vi "Lab Panel V6.00.vi"() -> ()   [LabVIEW 2017] (continued)
                            n2540 = Build Array(w4644) -> (w4630:dbl[])
                            n2541 = Build Array(w4639) -> (w4635:dbl[])
                            n2542 = Build Array(w4637) -> (w4634:dbl[])
                            n2543 = Build Array(w4642) -> (w4629:dbl[])
                            n2544 = Build Array("AMPS ON", "AMPS OFF", "VOLTS", "PF", "TEMP Live", "TEMP Neut", "CYCLE") -> (w4612:string[])
                            n2545 = Bundle By Name("Y"=w4635, "t0"=w4628) -> (w4627:waveform(dbl))  [unwired: 1 in]
                            n2546 = Bundle By Name("Y"=w4634, "t0"=w4628) -> (w4626:waveform(dbl))  [unwired: 1 in]
                            n2547 = Bundle By Name("Y"=w4633, "t0"=w4628) -> (w4625:waveform(dbl))  [unwired: 1 in]
                            n2548 = Bundle By Name("Y"=w4632, "t0"=w4628) -> (w4624:waveform(dbl))  [unwired: 1 in]
                            n2549 = Bundle By Name("Y"=w4631, "t0"=w4628) -> (w4623:waveform(dbl))  [unwired: 1 in]
                            n2550 = Bundle By Name("Y"=w4630, "t0"=w4628) -> (w4622:waveform(dbl))  [unwired: 1 in]
                            n2551 = Bundle By Name("Y"=w4629, "t0"=w4628) -> (w4621:waveform(dbl))  [unwired: 1 in]
                            n2552 = Build Array(w4627, w4626, w4625, w4624, w4623, w4622, w4621) -> (w4620:waveform(dbl)[])
                            n2553 = TDMS Write(0:w4641, 5:"TEST VALUES", 7:w4612, 9:w4620) -> (4:w4611:refnum<k34>, 6:w4610:string, 15:w4609:errorcluster)  [unwired: 2 in, 1 out]
                            n2554 = TDMS Write(0:w4611, 5:w4610, 7:"TIME", 9:w4607, 11:w4609) -> (15:w4606:errorcluster)  [unwired: 1 in, 3 out]
                            n2555 = local write "data file error"(w4606) -> ()
                          }
                        }
                      }
                    }
                  }
                }
              }
              frame #8 {
                n2556 = case shown="True" w4645 {
                  tunnel: w4649 -> [_ w4654]
                  tunnel: w4648 -> [_ w4653]
                  tunnel: w4647 -> [_ w4651]
                  tunnel: w4646 -> [_ w4650]
                  frame False {
                  }
                  frame True {
                    n2557 = local read "DISP LAB05-1"() -> (w4655:T4)
                    n2558 = local read "SIG LAB05-1"() -> (w4656:T2)
                    n2559 = local read "ON L05-1"() -> (w4652:cluster{"amps":dbl, "volts":dbl, "pf":dbl})
                    n2560 = Unbundle(w4656) -> ("AMPS"=w4662:dbl, "VOLTS"=w4660:dbl, "PF"=w4659:dbl, "Tmp Live"=w4658:dbl, "Tmp Neut"=w4661:dbl)
                    n2561 = Unbundle(w4655) -> ("CYCLE"=w4657:dbl)  [unwired: 2 out]
                    n2562 = stacked-sequence {
                      tunnel: w4662 -> [w4666 w4685]
                      tunnel: w4661 -> [_ w4684]
                      tunnel: w4660 -> [w4665 w4683]
                      tunnel: w4659 -> [w4664 w4682]
                      tunnel: w4658 -> [_ w4681]
                      tunnel: w4657 -> [_ w4680]
                      tunnel: w4654 -> [_ w4679]
                      tunnel: w4653 -> [w4667 _]
                      tunnel: w4652 -> [w4663 w4677]
                      tunnel: w4651 -> [_ w4678]
                      tunnel: w4650 -> [_ w4673]
                      frame #0 {
                        n2563 = case shown="True" w4667 {
                          tunnel: w4666 -> [_ w4672]
                          tunnel: w4665 -> [_ w4671]
                          tunnel: w4664 -> [_ w4670]
                          tunnel: w4663 -> [_ w4668]
                          frame False {
                          }
                          frame True {
                            n2564 = Bundle(cluster=w4668, "amps"=w4672, "volts"=w4671, "pf"=w4670) -> (w4669:cluster{"amps":dbl, "volts":dbl, "pf":dbl})
                            n2565 = local write "ON L05-1"(w4669) -> ()
                          }
                        }
                      }
                      frame #1 {
                        n2566 = Unbundle(w4677) -> ("amps"=w4676:dbl, "volts"=w4675:dbl, "pf"=w4674:dbl)
                        n2567 = case shown="True" w4678 {
                          tunnel: w4685 -> [_ w4717]
                          tunnel: w4684 -> [_ w4724]
                          tunnel: w4683 -> [_ _]
                          tunnel: w4682 -> [_ _]
                          tunnel: w4681 -> [_ w4723]
                          tunnel: w4680 -> [_ w4722]
                          tunnel: w4679 -> [_ w4687]
                          tunnel: w4676 -> [_ w4719]
                          tunnel: w4675 -> [_ w4718]
                          tunnel: w4674 -> [_ w4716]
                          tunnel: w4673 -> [_ w4708]
                          frame False {
                          }
                          frame True {
                            n2568 = local read "TDMS LAB05-1"() -> (w4721:refnum<k34>)
                            n2569 = Build Array(w4718) -> (w4713:dbl[])
                            n2570 = Build Array(w4716) -> (w4712:dbl[])
                            n2571 = Build Array(w4723) -> (w4711:dbl[])
                            n2572 = Build Array(w4724) -> (w4710:dbl[])
                            n2573 = Build Array(w4719) -> (w4715:dbl[])
                            n2574 = Build Array(w4717) -> (w4714:dbl[])
                            n2575 = Build Array(w4722) -> (w4709:dbl[])
                            n2576 = Build Array("AMPS ON", "AMPS OFF", "VOLTS", "PF", "TEMP Live", "TEMP Neut", "CYCLE") -> (w4692:string[])
                            n2577 = Bundle By Name("Y"=w4715, "t0"=w4708) -> (w4707:waveform(dbl))  [unwired: 1 in]
                            n2578 = Bundle By Name("Y"=w4714, "t0"=w4708) -> (w4706:waveform(dbl))  [unwired: 1 in]
                            n2579 = Bundle By Name("Y"=w4713, "t0"=w4708) -> (w4705:waveform(dbl))  [unwired: 1 in]
                            n2580 = Bundle By Name("Y"=w4712, "t0"=w4708) -> (w4704:waveform(dbl))  [unwired: 1 in]
                            n2581 = Bundle By Name("Y"=w4711, "t0"=w4708) -> (w4703:waveform(dbl))  [unwired: 1 in]
                            n2582 = Bundle By Name("Y"=w4710, "t0"=w4708) -> (w4702:waveform(dbl))  [unwired: 1 in]
                            n2583 = Bundle By Name("Y"=w4709, "t0"=w4708) -> (w4701:waveform(dbl))  [unwired: 1 in]
                            n2584 = Build Array(w4707, w4706, w4705, w4704, w4703, w4702, w4701) -> (w4700:waveform(dbl)[])
                            n2585 = TDMS Write(0:w4721, 5:"TEST VALUES", 7:w4692, 9:w4700) -> (4:w4691:refnum<k34>, 6:w4690:string, 15:w4689:errorcluster)  [unwired: 2 in, 1 out]
                            n2586 = TDMS Write(0:w4691, 5:w4690, 7:"TIME", 9:w4687, 11:w4689) -> (15:w4686:errorcluster)  [unwired: 1 in, 3 out]
                            n2587 = local write "data file error"(w4686) -> ()
                          }
                        }
                      }
                    }
                  }
                }
              }
              frame #9 {
                n2588 = case shown="True" w4725 {
                  tunnel: w4729 -> [_ w4734]
                  tunnel: w4728 -> [_ w4733]
                  tunnel: w4727 -> [_ w4731]
                  tunnel: w4726 -> [_ w4730]
                  frame False {
                  }
                  frame True {
                    n2589 = local read "DISP LAB05-2"() -> (w4735:T4)
                    n2590 = local read "SIG LAB05-2"() -> (w4736:T2)
                    n2591 = local read "ON L05-2"() -> (w4732:cluster{"amps":dbl, "volts":dbl, "pf":dbl})
                    n2592 = Unbundle(w4736) -> ("AMPS"=w4742:dbl, "VOLTS"=w4740:dbl, "PF"=w4739:dbl, "Tmp Live"=w4738:dbl, "Tmp Neut"=w4741:dbl)
                    n2593 = Unbundle(w4735) -> ("CYCLE"=w4737:dbl)  [unwired: 2 out]
                    n2594 = stacked-sequence {
                      tunnel: w4742 -> [w4746 w4765]
                      tunnel: w4741 -> [_ w4764]
                      tunnel: w4740 -> [w4745 w4763]
                      tunnel: w4739 -> [w4744 w4762]
                      tunnel: w4738 -> [_ w4761]
                      tunnel: w4737 -> [_ w4760]
                      tunnel: w4734 -> [_ w4759]
                      tunnel: w4733 -> [w4747 _]
                      tunnel: w4732 -> [w4743 w4757]
                      tunnel: w4731 -> [_ w4758]
                      tunnel: w4730 -> [_ w4753]
                      frame #0 {
                        n2595 = case shown="True" w4747 {
                          tunnel: w4746 -> [_ w4752]
                          tunnel: w4745 -> [_ w4751]
                          tunnel: w4744 -> [_ w4750]
                          tunnel: w4743 -> [_ w4748]
                          frame False {
                          }
                          frame True {
                            n2596 = Bundle(cluster=w4748, "amps"=w4752, "volts"=w4751, "pf"=w4750) -> (w4749:cluster{"amps":dbl, "volts":dbl, "pf":dbl})
                            n2597 = local write "ON L05-2"(w4749) -> ()
                          }
                        }
                      }
                      frame #1 {
                        n2598 = Unbundle(w4757) -> ("amps"=w4756:dbl, "volts"=w4755:dbl, "pf"=w4754:dbl)
                        n2599 = case shown="True" w4758 {
                          tunnel: w4765 -> [_ w4797]
                          tunnel: w4764 -> [_ w4804]
                          tunnel: w4763 -> [_ _]
                          tunnel: w4762 -> [_ _]
                          tunnel: w4761 -> [_ w4803]
                          tunnel: w4760 -> [_ w4802]
                          tunnel: w4759 -> [_ w4767]
                          tunnel: w4756 -> [_ w4799]
                          tunnel: w4755 -> [_ w4798]
                          tunnel: w4754 -> [_ w4796]
                          tunnel: w4753 -> [_ w4788]
                          frame False {
                          }
                          frame True {
                            n2600 = local read "TDMS LAB05-2"() -> (w4801:refnum<k34>)
                            n2601 = Build Array(w4798) -> (w4793:dbl[])
                            n2602 = Build Array(w4796) -> (w4792:dbl[])
                            n2603 = Build Array(w4803) -> (w4791:dbl[])
                            n2604 = Build Array(w4804) -> (w4790:dbl[])
                            n2605 = Build Array(w4799) -> (w4795:dbl[])
                            n2606 = Build Array(w4797) -> (w4794:dbl[])
                            n2607 = Build Array(w4802) -> (w4789:dbl[])
                            n2608 = Build Array("AMPS ON", "AMPS OFF", "VOLTS", "PF", "TEMP Live", "TEMP Neut", "CYCLE") -> (w4772:string[])
                            n2609 = Bundle By Name("Y"=w4795, "t0"=w4788) -> (w4787:waveform(dbl))  [unwired: 1 in]
                            n2610 = Bundle By Name("Y"=w4794, "t0"=w4788) -> (w4786:waveform(dbl))  [unwired: 1 in]
                            n2611 = Bundle By Name("Y"=w4793, "t0"=w4788) -> (w4785:waveform(dbl))  [unwired: 1 in]
                            n2612 = Bundle By Name("Y"=w4792, "t0"=w4788) -> (w4784:waveform(dbl))  [unwired: 1 in]
                            n2613 = Bundle By Name("Y"=w4791, "t0"=w4788) -> (w4783:waveform(dbl))  [unwired: 1 in]
                            n2614 = Bundle By Name("Y"=w4790, "t0"=w4788) -> (w4782:waveform(dbl))  [unwired: 1 in]
                            n2615 = Bundle By Name("Y"=w4789, "t0"=w4788) -> (w4781:waveform(dbl))  [unwired: 1 in]
                            n2616 = Build Array(w4787, w4786, w4785, w4784, w4783, w4782, w4781) -> (w4780:waveform(dbl)[])
                            n2617 = TDMS Write(0:w4801, 5:"TEST VALUES", 7:w4772, 9:w4780) -> (4:w4771:refnum<k34>, 6:w4770:string, 15:w4769:errorcluster)  [unwired: 2 in, 1 out]
                            n2618 = TDMS Write(0:w4771, 5:w4770, 7:"TIME", 9:w4767, 11:w4769) -> (15:w4766:errorcluster)  [unwired: 1 in, 3 out]
                            n2619 = local write "data file error"(w4766) -> ()
                          }
                        }
                      }
                    }
                  }
                }
              }
            }
          }
          frame #15 {
            # "display test values on chart"
            n2620 = local read "jig cycle"() -> (w4809:dbl)
            n2621 = local read "on loops"() -> (w4811:dbl)
            n2622 = Add(x=w4811, y=4) -> (x+y=w4808:dbl)
            n2623 = Equal?(x=w4809, y=3) -> (x = y?=w4807:bool)
            n2624 = Equal?(x=w4809, y=w4808) -> (x = y?=w4806:bool)
            n2625 = Or(x=w4807, y=w4806) -> (x .or. y?=w4805:bool)
            "graph flag" <- w4805
            n2626 = global write "Global display 3.vi" "graph flag"(w4805) -> ()
            n2627 = case shown="True" w4805 {
              frame False {
              }
              frame True {
                n2628 = local read "SIG LAB05-1"() -> (w4854:T2)
                n2629 = local read "SIG LAB04-2"() -> (w4855:T2)
                n2630 = local read "SIG LAB05-2"() -> (w4853:T2)
                n2631 = local read "SIG LAB04-1"() -> (w4856:T2)
                n2632 = local read "SIG LAB01-1"() -> (w4862:T2)
                n2633 = local read "SIG LAB03-1"() -> (w4858:T2)
                n2634 = local read "SIG LAB03-2"() -> (w4857:T2)
                n2635 = local read "SIG LAB02-2"() -> (w4859:T2)
                n2636 = local read "SIG LAB02-1"() -> (w4860:T2)
                n2637 = local read "SIG LAB01-2"() -> (w4861:T2)
                n2638 = Unbundle By Name(w4862) -> ("AMPS"=w4852:dbl, "VOLTS"=w4842:dbl, "Tmp Live"=w4832:dbl, "Tmp Neut"=w4822:dbl)
                n2639 = Unbundle(w4855) -> ("AMPS"=w4845:dbl, "VOLTS"=w4835:dbl, "Tmp Live"=w4825:dbl, "Tmp Neut"=w4815:dbl)  [unwired: 1 out]
                n2640 = Unbundle(w4854) -> ("AMPS"=w4844:dbl, "VOLTS"=w4834:dbl, "Tmp Live"=w4824:dbl, "Tmp Neut"=w4814:dbl)  [unwired: 1 out]
                n2641 = Unbundle(w4853) -> ("AMPS"=w4843:dbl, "VOLTS"=w4833:dbl, "Tmp Live"=w4823:dbl, "Tmp Neut"=w4813:dbl)  [unwired: 1 out]
                n2642 = Unbundle(w4856) -> ("AMPS"=w4846:dbl, "VOLTS"=w4836:dbl, "Tmp Live"=w4826:dbl, "Tmp Neut"=w4816:dbl)  [unwired: 1 out]
                n2643 = Unbundle(w4857) -> ("AMPS"=w4847:dbl, "VOLTS"=w4837:dbl, "Tmp Live"=w4827:dbl, "Tmp Neut"=w4817:dbl)  [unwired: 1 out]
                n2644 = Unbundle(w4858) -> ("AMPS"=w4848:dbl, "VOLTS"=w4838:dbl, "Tmp Live"=w4828:dbl, "Tmp Neut"=w4818:dbl)  [unwired: 1 out]
                n2645 = Unbundle(w4859) -> ("AMPS"=w4849:dbl, "VOLTS"=w4839:dbl, "Tmp Live"=w4829:dbl, "Tmp Neut"=w4819:dbl)  [unwired: 1 out]
                n2646 = Unbundle(w4860) -> ("AMPS"=w4850:dbl, "VOLTS"=w4840:dbl, "Tmp Live"=w4830:dbl, "Tmp Neut"=w4820:dbl)  [unwired: 1 out]
                n2647 = Unbundle(w4861) -> ("AMPS"=w4851:dbl, "VOLTS"=w4841:dbl, "Tmp Live"=w4831:dbl, "Tmp Neut"=w4821:dbl)  [unwired: 1 out]
                n2648 = stacked-sequence {
                  tunnel: w4852 -> [w4894 _ _]
                  tunnel: w4851 -> [w4893 _ _]
                  tunnel: w4850 -> [w4884 _ _]
                  tunnel: w4849 -> [w4883 _ _]
                  tunnel: w4848 -> [w4873 _ _]
                  tunnel: w4847 -> [w4872 _ _]
                  tunnel: w4846 -> [_ w4917 _]
                  tunnel: w4845 -> [_ w4916 _]
                  tunnel: w4844 -> [_ w4906 _]
                  tunnel: w4843 -> [_ w4905 _]
                  tunnel: w4842 -> [w4891 _ _]
                  tunnel: w4841 -> [w4890 _ _]
                  tunnel: w4840 -> [w4881 _ _]
                  tunnel: w4839 -> [w4880 _ _]
                  tunnel: w4838 -> [w4871 _ _]
                  tunnel: w4837 -> [w4870 _ _]
                  tunnel: w4836 -> [_ w4915 _]
                  tunnel: w4835 -> [_ w4914 _]
                  tunnel: w4834 -> [_ w4904 _]
                  tunnel: w4833 -> [_ w4903 _]
                  tunnel: w4832 -> [w4888 _ _]
                  tunnel: w4831 -> [w4886 _ _]
                  tunnel: w4830 -> [w4877 _ _]
                  tunnel: w4829 -> [w4875 _ _]
                  tunnel: w4828 -> [w4869 _ _]
                  tunnel: w4827 -> [w4867 _ _]
                  tunnel: w4826 -> [_ w4913 _]
                  tunnel: w4825 -> [_ w4911 _]
                  tunnel: w4824 -> [_ w4902 _]
                  tunnel: w4823 -> [_ w4900 _]
                  tunnel: w4822 -> [w4887 _ _]
                  tunnel: w4821 -> [w4885 _ _]
                  tunnel: w4820 -> [w4876 _ _]
                  tunnel: w4819 -> [w4874 _ _]
                  tunnel: w4818 -> [w4868 _ _]
                  tunnel: w4817 -> [w4866 _ _]
                  tunnel: w4816 -> [_ w4912 _]
                  tunnel: w4815 -> [_ w4910 _]
                  tunnel: w4814 -> [_ w4901 _]
                  tunnel: w4813 -> [_ w4899 _]
                  frame #0 {
                    n2649 = Merge Signals(w4894, w4893) -> (→"LAB01 AMPS":dynamicdata)
                    n2650 = Merge Signals(w4891, w4890) -> (→"LAB01 VOLTS":dynamicdata)
                    n2651 = Merge Signals(w4871, w4870) -> (→"LAB03 VOLTS":dynamicdata)
                    n2652 = Merge Signals(w4888, w4887, w4886, w4885) -> (→"LAB01 deg C":dynamicdata)
                    n2653 = Merge Signals(w4884, w4883) -> (→"LAB02 AMPS":dynamicdata)
                    n2654 = Merge Signals(w4877, w4876, w4875, w4874) -> (→"LAB02 deg C":dynamicdata)
                    n2655 = Merge Signals(w4869, w4868, w4867, w4866) -> (→"LAB03 deg C":dynamicdata)
                    n2656 = Merge Signals(w4881, w4880) -> (→"LAB02 VOLTS":dynamicdata)
                    n2657 = Merge Signals(w4873, w4872) -> (→"LAB03 AMPS":dynamicdata)
                  }
                  frame #1 {
                    n2658 = Merge Signals(w4904, w4903) -> (→"LAB05 VOLTS":dynamicdata)
                    n2659 = Merge Signals(w4917, w4916) -> (→"LAB04 AMPS":dynamicdata)
                    n2660 = Merge Signals(w4906, w4905) -> (→"LAB05 AMPS":dynamicdata)
                    n2661 = Merge Signals(w4902, w4901, w4900, w4899) -> (→"LAB05 deg C":dynamicdata)
                    n2662 = Merge Signals(w4913, w4912, w4911, w4910) -> (→"LAB04 deg C":dynamicdata)
                    n2663 = Merge Signals(w4915, w4914) -> (→"LAB04 VOLTS":dynamicdata)
                  }
                  frame #2 {
                    n2664 = local read "LAB05 VOLTS"() -> (w4925:dynamicdata)
                    n2665 = local read "LAB04 VOLTS"() -> (w4926:dynamicdata)
                    n2666 = local read "LAB05 AMPS"() -> (w4931:dynamicdata)
                    n2667 = local read "LAB02 VOLTS"() -> (w4928:dynamicdata)
                    n2668 = local read "LAB03 VOLTS"() -> (w4927:dynamicdata)
                    n2669 = local read "LAB01 VOLTS"() -> (w4929:dynamicdata)
                    n2670 = local read "LAB04 AMPS"() -> (w4932:dynamicdata)
                    n2671 = local read "LAB03 AMPS"() -> (w4933:dynamicdata)
                    n2672 = local read "LAB03 deg C"() -> (w4921:dynamicdata)
                    n2673 = local read "LAB02 AMPS"() -> (w4934:dynamicdata)
                    n2674 = local read "LAB04 deg C"() -> (w4920:dynamicdata)
                    n2675 = local read "LAB05 deg C"() -> (w4919:dynamicdata)
                    n2676 = local read "LAB02 deg C"() -> (w4922:dynamicdata)
                    n2677 = local read "LAB01 deg C"() -> (w4923:dynamicdata)
                    n2678 = local read "LAB01 AMPS"() -> (w4935:dynamicdata)
                    n2679 = Merge Signals(w4923, w4922, w4921, w4920, w4919) -> (w4918:dynamicdata)
                    n2680 = Merge Signals(w4935, w4934, w4933, w4932, w4931) -> (w4930:dynamicdata)
                    n2681 = Merge Signals(w4929, w4928, w4927, w4926, w4925) -> (w4924:dynamicdata)
                    n2682 = global write "Global display 3.vi" "graph volts"(w4924) -> ()
                    n2683 = global write "Global display 3.vi" "graph deg C"(w4918) -> ()
                    n2684 = global write "Global display 3.vi" "graph amps"(w4930) -> ()
                  }
                }
              }
            }
          }
          frame #16 {
            # "check for amps fail"
            # "check for cycle test & temperature rise fail conditions"
            n2685 = local read "on loops"() -> (w4962:dbl)
            n2686 = local read "jig cycle"() -> (w4959:dbl)
            n2687 = Add(x=w4962, y=5.0) -> (x+y=w4960:dbl)
            n2688 = Equal?(x=w4959, y=w4960) -> (x = y?=w4955:bool)
            n2689 = local read "jig cycle"() -> (w4964:dbl)
            n2690 = Equal?(x=w4964, y=3.0) -> (x = y?=w4957:bool)
            n2691 = local read "Fail Loops"() -> (w4936:dbl)
            n2692 = stacked-sequence {
              tunnel: w4958 -> [w4967 _ _ _ _ _ _ _ _ _]
              tunnel: w4957 -> [w4968 w4988 w5008 w5028 w5048 w5068 w5088 w5108 w5128 w5148]
              tunnel: w4956 -> [w4965 _ _ _ _ _ _ _ _ _]
              tunnel: w4955 -> [w4966 w4987 w5007 w5027 w5047 w5067 w5087 w5107 w5127 w5147]
              tunnel: w4954 -> [_ w4986 _ _ _ _ _ _ _ _]
              tunnel: w4953 -> [_ w4985 _ _ _ _ _ _ _ _]
              tunnel: w4952 -> [_ _ w5006 _ _ _ _ _ _ _]
              tunnel: w4951 -> [_ _ w5005 _ _ _ _ _ _ _]
              tunnel: w4950 -> [_ _ _ w5026 _ _ _ _ _ _]
              tunnel: w4949 -> [_ _ _ w5025 _ _ _ _ _ _]
              tunnel: w4948 -> [_ _ _ _ w5046 _ _ _ _ _]
              tunnel: w4947 -> [_ _ _ _ w5045 _ _ _ _ _]
              tunnel: w4946 -> [_ _ _ _ _ w5066 _ _ _ _]
              tunnel: w4945 -> [_ _ _ _ _ w5065 _ _ _ _]
              tunnel: w4944 -> [_ _ _ _ _ _ w5086 _ _ _]
              tunnel: w4943 -> [_ _ _ _ _ _ w5085 _ _ _]
              tunnel: w4942 -> [_ _ _ _ _ _ _ w5106 _ _]
              tunnel: w4941 -> [_ _ _ _ _ _ _ w5105 _ _]
              tunnel: w4940 -> [_ _ _ _ _ _ _ _ w5126 _]
              tunnel: w4939 -> [_ _ _ _ _ _ _ _ w5125 _]
              tunnel: w4938 -> [_ _ _ _ _ _ _ _ _ w5146]
              tunnel: w4937 -> [_ _ _ _ _ _ _ _ _ w5145]
              frame #0 {
                # "LAB01-1"
                n2693 = case shown="True" w4965 {
                  tunnel: w4968 -> [_ w4981]
                  tunnel: w4967 -> [_ w4978]
                  tunnel: w4966 -> [_ w4977]
                  frame False {
                  }
                  frame True {
                    n2694 = local read "TEMP START LAB01-1"() -> (w4983:cluster{"TL":dbl, "TN":dbl})
                    n2695 = local read "RESULT LAB01-1"() -> (w4972:bool)
                    n2696 = local read "FAIL LAB01-1"() -> (w4975:cluster{"LO":dbl, "HI":dbl})
                    n2697 = local read "TDMS LAB01-1"() -> (w4982:refnum<k34>)
                    n2698 = local read "SET LAB01-1"() -> (w4979:T6)
                    n2699 = local read "DISP LAB01-1"() -> (w4980:T4)
                    n2700 = local read "SIG LAB01-1"() -> (w4984:T2)
                    n2701 = Bundle("FAIL LAB01-1"=w4975, "SIG LAB01-1"=w4984, "TEMP START LAB01-1"=w4983, "DISP LAB01-1"=w4980, "SET LAB01-1"=w4979, "TDMS LAB01-1"=w4982) -> (w4969:T36)  [unwired: 1 in]
                    n2702 = call "sub vi - cycle&temp fail v7.vi"("Amps Lo?"=w4981, "Input Cluster"=w4969, "SELECT"=w4978, "Amps Hi?"=w4977, "Result In"=w4972) -> ("(FAIL) out"=w4974:cluster{"FAIL LO":dbl, "FAIL HI":dbl}, "(DISP) out"=w4970:T4, "T-RISE"=w4971:cluster{"T-RISE (L)":dbl, "T-RISE (N)":dbl}, "Result Out"=w4973:bool, "file error"=w4976:errorcluster)  [unwired: 10 in]
                    n2703 = local write "TEMP RISE LAB01-1"(w4971) -> ()
                    n2704 = local write "FAIL LAB01-1"(w4974) -> ()
                    n2705 = local write "DISP LAB01-1"(w4970) -> ()
                    n2706 = local write "RESULT LAB01-1"(w4973) -> ()
                    n2707 = local write "data file error"(w4976) -> ()
                  }
                }
              }
              frame #1 {
                # "LAB01-2"
                n2708 = case shown="True" w4986 {
                  tunnel: w4988 -> [_ w5001]
                  tunnel: w4985 -> [_ w4998]
                  tunnel: w4987 -> [_ w4997]
                  frame False {
                  }
                  frame True {
                    n2709 = local read "TEMP START LAB01-2"() -> (w5003:cluster{"TL":dbl, "TN":dbl})
                    n2710 = local read "FAIL LAB01-2"() -> (w4994:cluster{"LO":dbl, "HI":dbl})
                    n2711 = local read "TDMS LAB01-2"() -> (w5002:refnum<k34>)
                    n2712 = local read "SET LAB01-2"() -> (w4999:T5)
                    n2713 = local read "DISP LAB01-2"() -> (w5000:T4)
                    n2714 = local read "RESULT LAB01-2"() -> (w4991:bool)
                    n2715 = local read "SIG LAB01-2"() -> (w5004:T2)
                    n2716 = Bundle("FAIL LAB01-2"=w4994, "SIG LAB01-2"=w5004, "TEMP START LAB01-2"=w5003, "DISP LAB01-2"=w5000, "SET LAB01-2"=w4999, "TDMS LAB01-2"=w5002) -> (w4989:T37)  [unwired: 1 in]
                    n2717 = call "sub vi - cycle&temp fail v7.vi"("Amps Lo?"=w5001, "Input Cluster"=w4989, "SELECT"=w4998, "Amps Hi?"=w4997, "Result In"=w4991) -> ("(FAIL) out"=w4993:cluster{"FAIL LO":dbl, "FAIL HI":dbl}, "(DISP) out"=w4996:T4, "T-RISE"=w4990:cluster{"T-RISE (L)":dbl, "T-RISE (N)":dbl}, "Result Out"=w4992:bool, "file error"=w4995:errorcluster)  [unwired: 10 in]
                    n2718 = local write "TEMP RISE LAB01-2"(w4990) -> ()
                    n2719 = local write "FAIL LAB01-2"(w4993) -> ()
                    n2720 = local write "DISP LAB01-2"(w4996) -> ()
                    n2721 = local write "RESULT LAB01-2"(w4992) -> ()
                    n2722 = local write "data file error"(w4995) -> ()
                  }
                }
              }
              frame #2 {
                # "LAB02-1"
                n2723 = case shown="True" w5006 {
                  tunnel: w5008 -> [_ w5021]
                  tunnel: w5005 -> [_ w5018]
                  tunnel: w5007 -> [_ w5017]
                  frame False {
                  }
                  frame True {
                    n2724 = local read "TEMP START LAB02-1"() -> (w5023:cluster{"TL":dbl, "TN":dbl})
                    n2725 = local read "FAIL LAB02-1"() -> (w5014:cluster{"LO":dbl, "HI":dbl})
                    n2726 = local read "TDMS LAB02-1"() -> (w5022:refnum<k34>)
                    n2727 = local read "SET LAB02-1"() -> (w5019:T5)
                    n2728 = local read "DISP LAB02-1"() -> (w5020:T4)
                    n2729 = local read "SIG LAB02-1"() -> (w5024:T2)
                    n2730 = local read "RESULT LAB02-1"() -> (w5011:bool)
                    n2731 = Bundle("FAIL LAB02-1"=w5014, "SIG LAB02-1"=w5024, "TEMP START LAB02-1"=w5023, "DISP LAB02-1"=w5020, "SET LAB02-1"=w5019, "TDMS LAB02-1"=w5022) -> (w5009:T38)  [unwired: 1 in]
                    n2732 = call "sub vi - cycle&temp fail v7.vi"("Amps Lo?"=w5021, "Input Cluster"=w5009, "SELECT"=w5018, "Amps Hi?"=w5017, "Result In"=w5011) -> ("(FAIL) out"=w5013:cluster{"FAIL LO":dbl, "FAIL HI":dbl}, "(DISP) out"=w5016:T4, "T-RISE"=w5010:cluster{"T-RISE (L)":dbl, "T-RISE (N)":dbl}, "Result Out"=w5012:bool, "file error"=w5015:errorcluster)  [unwired: 10 in]
                    n2733 = local write "TEMP RISE LAB02-1"(w5010) -> ()
                    n2734 = local write "FAIL LAB02-1"(w5013) -> ()
                    n2735 = local write "DISP LAB02-1"(w5016) -> ()
                    n2736 = local write "RESULT LAB02-1"(w5012) -> ()
                    n2737 = local write "data file error"(w5015) -> ()
                  }
                }
              }
              frame #3 {
                # "LAB02-2"
                n2738 = case shown="True" w5026 {
                  tunnel: w5028 -> [_ w5041]
                  tunnel: w5025 -> [_ w5038]
                  tunnel: w5027 -> [_ w5037]
                  frame False {
                  }
                  frame True {
                    n2739 = local read "TEMP START LAB02-2"() -> (w5043:cluster{"TL":dbl, "TN":dbl})
                    n2740 = local read "FAIL LAB02-2"() -> (w5034:cluster{"LO":dbl, "HI":dbl})
                    n2741 = local read "TDMS LAB02-2"() -> (w5042:refnum<k34>)
                    n2742 = local read "SET LAB02-2"() -> (w5039:T5)
                    n2743 = local read "DISP LAB02-2"() -> (w5040:T4)
                    n2744 = local read "SIG LAB02-2"() -> (w5044:T2)
                    n2745 = local read "RESULT LAB02-2"() -> (w5031:bool)
                    n2746 = Bundle("FAIL LAB02-2"=w5034, "SIG LAB02-2"=w5044, "TEMP START LAB02-2"=w5043, "DISP LAB02-2"=w5040, "SET LAB02-2"=w5039, "TDMS LAB02-2"=w5042) -> (w5029:T39)  [unwired: 1 in]
                    n2747 = call "sub vi - cycle&temp fail v7.vi"("Amps Lo?"=w5041, "Input Cluster"=w5029, "SELECT"=w5038, "Amps Hi?"=w5037, "Result In"=w5031) -> ("(FAIL) out"=w5033:cluster{"FAIL LO":dbl, "FAIL HI":dbl}, "(DISP) out"=w5036:T4, "T-RISE"=w5030:cluster{"T-RISE (L)":dbl, "T-RISE (N)":dbl}, "Result Out"=w5032:bool, "file error"=w5035:errorcluster)  [unwired: 10 in]
                    n2748 = local write "TEMP RISE LAB02-2"(w5030) -> ()
                    n2749 = local write "FAIL LAB02-2"(w5033) -> ()
                    n2750 = local write "DISP LAB02-2"(w5036) -> ()
                    n2751 = local write "RESULT LAB02-2"(w5032) -> ()
                    n2752 = local write "data file error"(w5035) -> ()
                  }
                }
              }
              frame #4 {
                # "LAB03-1"
                n2753 = case shown="True" w5046 {
                  tunnel: w5048 -> [_ w5061]
                  tunnel: w5045 -> [_ w5058]
                  tunnel: w5047 -> [_ w5057]
                  frame False {
                  }
                  frame True {
                    n2754 = local read "TEMP START LAB03-1"() -> (w5063:cluster{"TL":dbl, "TN":dbl})
                    n2755 = local read "FAIL LAB03-1"() -> (w5054:cluster{"LO":dbl, "HI":dbl})
                    n2756 = local read "TDMS LAB03-1"() -> (w5062:refnum<k34>)
                    n2757 = local read "SET LAB03-1"() -> (w5059:T5)
                    n2758 = local read "DISP LAB03-1"() -> (w5060:T4)
                    n2759 = local read "SIG LAB03-1"() -> (w5064:T2)
                    n2760 = local read "RESULT LAB03-1"() -> (w5051:bool)
                    n2761 = Bundle("FAIL LAB03-1"=w5054, "SIG LAB03-1"=w5064, "TEMP START LAB03-1"=w5063, "DISP LAB03-1"=w5060, "SET LAB03-1"=w5059, "TDMS LAB03-1"=w5062) -> (w5049:T40)  [unwired: 1 in]
                    n2762 = call "sub vi - cycle&temp fail v7.vi"("Amps Lo?"=w5061, "Input Cluster"=w5049, "SELECT"=w5058, "Amps Hi?"=w5057, "Result In"=w5051) -> ("(FAIL) out"=w5053:cluster{"FAIL LO":dbl, "FAIL HI":dbl}, "(DISP) out"=w5056:T4, "T-RISE"=w5050:cluster{"T-RISE (L)":dbl, "T-RISE (N)":dbl}, "Result Out"=w5052:bool, "file error"=w5055:errorcluster)  [unwired: 10 in]
                    n2763 = local write "TEMP RISE LAB03-1"(w5050) -> ()
                    n2764 = local write "FAIL LAB03-1"(w5053) -> ()
                    n2765 = local write "DISP LAB03-1"(w5056) -> ()
                    n2766 = local write "RESULT LAB03-1"(w5052) -> ()
                    n2767 = local write "data file error"(w5055) -> ()
                  }
                }
              }
              frame #5 {
                # "LAB03-2"
                n2768 = case shown="True" w5066 {
                  tunnel: w5068 -> [_ w5081]
                  tunnel: w5065 -> [_ w5078]
                  tunnel: w5067 -> [_ w5077]
                  frame False {
                  }
                  frame True {
                    n2769 = local read "TEMP START LAB03-2"() -> (w5083:cluster{"TL":dbl, "TN":dbl})
                    n2770 = local read "FAIL LAB03-2"() -> (w5074:cluster{"LO":dbl, "HI":dbl})
                    n2771 = local read "TDMS LAB03-2"() -> (w5082:refnum<k34>)
                    n2772 = local read "SET LAB03-2"() -> (w5079:T5)
                    n2773 = local read "DISP LAB03-2"() -> (w5080:T4)
                    n2774 = local read "RESULT LAB03-2"() -> (w5071:bool)
                    n2775 = local read "SIG LAB03-2"() -> (w5084:T2)
                    n2776 = Bundle("FAIL LAB03-2"=w5074, "SIG LAB03-2"=w5084, "TEMP START LAB03-2"=w5083, "DISP LAB03-2"=w5080, "SET LAB03-2"=w5079, "TDMS LAB03-2"=w5082) -> (w5069:T41)  [unwired: 1 in]
                    n2777 = call "sub vi - cycle&temp fail v7.vi"("Amps Lo?"=w5081, "Input Cluster"=w5069, "SELECT"=w5078, "Amps Hi?"=w5077, "Result In"=w5071) -> ("(FAIL) out"=w5073:cluster{"FAIL LO":dbl, "FAIL HI":dbl}, "(DISP) out"=w5076:T4, "T-RISE"=w5070:cluster{"T-RISE (L)":dbl, "T-RISE (N)":dbl}, "Result Out"=w5072:bool, "file error"=w5075:errorcluster)  [unwired: 10 in]
                    n2778 = local write "FAIL LAB03-2"(w5073) -> ()
                    n2779 = local write "TEMP RISE LAB03-2"(w5070) -> ()
                    n2780 = local write "DISP LAB03-2"(w5076) -> ()
                    n2781 = local write "RESULT LAB03-2"(w5072) -> ()
                    n2782 = local write "data file error"(w5075) -> ()
                  }
                }
              }
              frame #6 {
                # "LAB04-1"
                n2783 = case shown="True" w5086 {
                  tunnel: w5088 -> [_ w5101]
                  tunnel: w5085 -> [_ w5098]
                  tunnel: w5087 -> [_ w5097]
                  frame False {
                  }
                  frame True {
                    n2784 = local read "TEMP START LAB04-1"() -> (w5103:cluster{"TL":dbl, "TN":dbl})
                    n2785 = local read "FAIL LAB04-1"() -> (w5094:cluster{"LO":dbl, "HI":dbl})
                    n2786 = local read "TDMS LAB04-1"() -> (w5102:refnum<k34>)
                    n2787 = local read "SET LAB04-1"() -> (w5099:T5)
                    n2788 = local read "DISP LAB04-1"() -> (w5100:T4)
                    n2789 = local read "SIG LAB04-1"() -> (w5104:T2)
                    n2790 = local read "RESULT LAB04-1"() -> (w5091:bool)
                    n2791 = Bundle("FAIL LAB04-1"=w5094, "SIG LAB04-1"=w5104, "TEMP START LAB04-1"=w5103, "DISP LAB04-1"=w5100, "SET LAB04-1"=w5099, "TDMS LAB04-1"=w5102) -> (w5089:T42)  [unwired: 1 in]
                    n2792 = call "sub vi - cycle&temp fail v7.vi"("Amps Lo?"=w5101, "Input Cluster"=w5089, "SELECT"=w5098, "Amps Hi?"=w5097, "Result In"=w5091) -> ("(FAIL) out"=w5093:cluster{"FAIL LO":dbl, "FAIL HI":dbl}, "(DISP) out"=w5096:T4, "T-RISE"=w5090:cluster{"T-RISE (L)":dbl, "T-RISE (N)":dbl}, "Result Out"=w5092:bool, "file error"=w5095:errorcluster)  [unwired: 10 in]
                    n2793 = local write "TEMP RISE LAB04-1"(w5090) -> ()
                    n2794 = local write "FAIL LAB04-1"(w5093) -> ()
                    n2795 = local write "DISP LAB04-1"(w5096) -> ()
                    n2796 = local write "RESULT LAB04-1"(w5092) -> ()
                    n2797 = local write "data file error"(w5095) -> ()
                  }
                }
              }
              frame #7 {
                # "LAB04-2"
                n2798 = case shown="True" w5106 {
                  tunnel: w5108 -> [_ w5121]
                  tunnel: w5105 -> [_ w5118]
                  tunnel: w5107 -> [_ w5117]
                  frame False {
                  }
                  frame True {
                    n2799 = local read "TEMP START LAB04-2"() -> (w5123:cluster{"TL":dbl, "TN":dbl})
                    n2800 = local read "FAIL LAB04-2"() -> (w5114:cluster{"LO":dbl, "HI":dbl})
                    n2801 = local read "TDMS LAB04-2"() -> (w5122:refnum<k34>)
                    n2802 = local read "SET LAB04-2"() -> (w5119:T5)
                    n2803 = local read "DISP LAB04-2"() -> (w5120:T4)
                    n2804 = local read "SIG LAB04-2"() -> (w5124:T2)
                    n2805 = local read "RESULT LAB04-2"() -> (w5111:bool)
                    n2806 = Bundle("FAIL LAB04-2"=w5114, "SIG LAB04-2"=w5124, "TEMP START LAB04-2"=w5123, "DISP LAB04-2"=w5120, "SET LAB04-2"=w5119, "TDMS LAB04-2"=w5122) -> (w5109:T43)  [unwired: 1 in]
                    n2807 = call "sub vi - cycle&temp fail v7.vi"("Amps Lo?"=w5121, "Input Cluster"=w5109, "SELECT"=w5118, "Amps Hi?"=w5117, "Result In"=w5111) -> ("(FAIL) out"=w5113:cluster{"FAIL LO":dbl, "FAIL HI":dbl}, "(DISP) out"=w5116:T4, "T-RISE"=w5110:cluster{"T-RISE (L)":dbl, "T-RISE (N)":dbl}, "Result Out"=w5112:bool, "file error"=w5115:errorcluster)  [unwired: 10 in]
                    n2808 = local write "TEMP RISE LAB04-2"(w5110) -> ()
                    n2809 = local write "FAIL LAB04-2"(w5113) -> ()
                    n2810 = local write "DISP LAB04-2"(w5116) -> ()
                    n2811 = local write "RESULT LAB04-2"(w5112) -> ()
                    n2812 = local write "data file error"(w5115) -> ()
                  }
                }
              }
              frame #8 {
                # "LAB05-1"
                n2813 = case shown="True" w5126 {
                  tunnel: w5128 -> [_ w5141]
                  tunnel: w5125 -> [_ w5138]
                  tunnel: w5127 -> [_ w5137]
                  frame False {
                  }
                  frame True {
                    n2814 = local read "TEMP START LAB05-1"() -> (w5143:cluster{"TL":dbl, "TN":dbl})
                    n2815 = local read "FAIL LAB05-1"() -> (w5134:cluster{"LO":dbl, "HI":dbl})
                    n2816 = local read "TDMS LAB05-1"() -> (w5142:refnum<k34>)
                    n2817 = local read "SET LAB05-1"() -> (w5139:T5)
                    n2818 = local read "DISP LAB05-1"() -> (w5140:T4)
                    n2819 = local read "SIG LAB05-1"() -> (w5144:T2)
                    n2820 = local read "RESULT LAB05-1"() -> (w5131:bool)
                    n2821 = Bundle("FAIL LAB05-1"=w5134, "SIG LAB05-1"=w5144, "TEMP START LAB05-1"=w5143, "DISP LAB05-1"=w5140, "SET LAB05-1"=w5139, "TDMS LAB05-1"=w5142) -> (w5129:T44)  [unwired: 1 in]
                    n2822 = call "sub vi - cycle&temp fail v7.vi"("Amps Lo?"=w5141, "Input Cluster"=w5129, "SELECT"=w5138, "Amps Hi?"=w5137, "Result In"=w5131) -> ("(FAIL) out"=w5133:cluster{"FAIL LO":dbl, "FAIL HI":dbl}, "(DISP) out"=w5136:T4, "T-RISE"=w5130:cluster{"T-RISE (L)":dbl, "T-RISE (N)":dbl}, "Result Out"=w5132:bool, "file error"=w5135:errorcluster)  [unwired: 10 in]
                    n2823 = local write "TEMP RISE LAB05-1"(w5130) -> ()
                    n2824 = local write "FAIL LAB05-1"(w5133) -> ()
                    n2825 = local write "DISP LAB05-1"(w5136) -> ()
                    n2826 = local write "RESULT LAB05-1"(w5132) -> ()
                    n2827 = local write "data file error"(w5135) -> ()
                  }
                }
              }
              frame #9 {
                # "LAB05-2"
                n2828 = case shown="True" w5146 {
                  tunnel: w5148 -> [_ w5161]
                  tunnel: w5145 -> [_ w5158]
                  tunnel: w5147 -> [_ w5157]
                  frame False {
                  }
                  frame True {
                    n2829 = local read "TEMP START LAB05-2"() -> (w5163:cluster{"TL":dbl, "TN":dbl})
                    n2830 = local read "FAIL LAB05-2"() -> (w5154:cluster{"LO":dbl, "HI":dbl})
                    n2831 = local read "TDMS LAB05-2"() -> (w5162:refnum<k34>)
                    n2832 = local read "SET LAB05-2"() -> (w5159:T5)
                    n2833 = local read "DISP LAB05-2"() -> (w5160:T4)
                    n2834 = local read "SIG LAB05-2"() -> (w5164:T2)
                    n2835 = local read "RESULT LAB05-2"() -> (w5151:bool)
                    n2836 = Bundle("FAIL LAB05-2"=w5154, "SIG LAB05-2"=w5164, "TEMP START LAB05-2"=w5163, "DISP LAB05-2"=w5160, "SET LAB05-2"=w5159, "TDMS LAB05-2"=w5162) -> (w5149:T45)  [unwired: 1 in]
                    n2837 = call "sub vi - cycle&temp fail v7.vi"("Amps Lo?"=w5161, "Input Cluster"=w5149, "SELECT"=w5158, "Amps Hi?"=w5157, "Result In"=w5151) -> ("(FAIL) out"=w5153:cluster{"FAIL LO":dbl, "FAIL HI":dbl}, "(DISP) out"=w5156:T4, "T-RISE"=w5150:cluster{"T-RISE (L)":dbl, "T-RISE (N)":dbl}, "Result Out"=w5152:bool, "file error"=w5155:errorcluster)  [unwired: 10 in]
                    n2838 = local write "TEMP RISE LAB05-2"(w5150) -> ()
                    n2839 = local write "FAIL LAB05-2"(w5153) -> ()
                    n2840 = local write "DISP LAB05-2"(w5156) -> ()
                    n2841 = local write "RESULT LAB05-2"(w5152) -> ()
                    n2842 = local write "data file error"(w5155) -> ()
                  }
                }
              }
            }
            n2843 = global write "Global 1.vi" "fail count"(w4936) -> ()
          }
          frame #17 {
            # "run calibration routine"
            n2844 = local read "SET (cal)"() -> (w5165:bool)
            n2845 = case shown="True" w5165 {
              frame False {
              }
              frame True {
                n2846 = stacked-sequence {
                  seq-local: [w5166 _ _] -> [_ w5168 _]
                  frame #0 {
                    n2847 = call "CALIBRATION PASSWORD"() -> ("PASSWORD"=w5166:string)  [unwired: 17 in, 2 out]
                  }
                  frame #1 {
                    n2848 = Equal?(x=w5168, y="7777") -> (x = y?=w5167:bool)
                    n2849 = case shown="True" w5167 {
                      frame False {
                      }
                      frame True {
                        n2850 = stacked-sequence {
                          frame #0 {
                            n2851 = local read "SAMPLES"() -> (w5170:dbl)
                            n2852 = local read "AI Task2"() -> (w5171:dbl)
                            n2853 = local read "AI Task1"() -> (w5172:dbl)
                            n2854 = local read "AI Task0"() -> (w5173:dbl)
                            n2855 = local read "Temp Test Cal"() -> (w5174:dbl)
                            n2856 = call "sub vi - calibration v2.vi"("Samples"=w5170, "Task2"=w5171, "Task1"=w5172, "Task0"=w5173, "Temp Test Cal"=w5174) -> ()  [unwired: 7 in]
                          }
                          frame #1 {
                            n2857 = call "sub vi - get calibration values v1.vi"() -> ("TEMP REF CAL"=w5175:dbl, "LAB01 (CAL)"=w5180:T15, "LAB02 (CAL)"=w5179:T16, "LAB03 (CAL)"=w5178:T15, "LAB04 (CAL)"=w5177:T15, "calibration file error out"=w5181:errorcluster, "LAB05 (CAL)"=w5176:T15)  [unwired: 9 in]
                            n2858 = local write "TEMP REF cal"(w5175) -> ()
                            n2859 = local write "cal file error out"(w5181) -> ()
                            n2860 = local write "CAL LAB04"(w5177) -> ()
                            n2861 = local write "CAL LAB05"(w5176) -> ()
                            n2862 = local write "CAL LAB01"(w5180) -> ()
                            n2863 = local write "CAL LAB02"(w5179) -> ()
                            n2864 = local write "CAL LAB03"(w5178) -> ()
                          }
                        }
                      }
                    }
                  }
                  frame #2 {
                    n2865 = local write "SET (cal)"(FALSE) -> ()
                  }
                }
              }
            }
          }
          frame #18 {
            # "save certain settings to file"
            n2866 = String To Path(string="c:\\crabtree\\Set Up\\") -> (path=w5184:path)
            n2867 = Build Path(base path=w5184, name or relative path="settings.bin") -> (appended path=w5186:path)
            n2868 = Build Path(base path=w5184, name or relative path="mail.bin") -> (appended path=w5183:path)
            n2869 = Create Folder(path (use dialog)=w5184) -> (error out=w5189:errorcluster)  [unwired: 2 in, 2 out]
            n2870 = call <vilib>:"Clear Errors.vi"("error in (no error)"=w5189) -> ()  [unwired: 5 in, 2 out]
            n2871 = stacked-sequence {
              seq-local: [w5201 _] -> [_ w5214]
              tunnel: w5186 -> [_ w5215]
              tunnel: w5183 -> [_ w5213]
              frame #0 {
                n2872 = local read "C drive data root dir"() -> (w5200:path)
                n2873 = local read "Select COM port"() -> (w5197:refnum<visa-resource-name>)
                n2874 = local read "Network Directory"() -> (w5206:path)
                n2875 = local read "SET LAB05-2"() -> (w5205:T5)
                n2876 = local read "SET LAB05-1"() -> (w5204:T5)
                n2877 = local read "SET LAB04-2"() -> (w5203:T5)
                n2878 = local read "SET LAB03-2"() -> (w5207:T5)
                n2879 = local read "SET LAB04-1"() -> (w5202:T5)
                n2880 = local read "SET LAB03-1"() -> (w5208:T5)
                n2881 = local read "SET LAB02-2"() -> (w5209:T5)
                n2882 = local read "SET LAB02-1"() -> (w5210:T5)
                n2883 = local read "SET LAB01-2"() -> (w5211:T5)
                n2884 = local read "SET LAB01-1"() -> (w5212:T6)
                n2885 = local read "Temp Delay Lps"() -> (w5196:dbl)
                n2886 = local read "Amps Fail level"() -> (w5192:dbl)
                n2887 = local read "Temp Test Cal"() -> (w5193:dbl)
                n2888 = local read "Temp Value"() -> (w5195:dbl)
                n2889 = local read "Mail Test File To:"() -> (w5191:string)
                n2890 = local read "Fail Loops"() -> (w5194:dbl)
                n2891 = local read "Mail Test Fail"() -> (w5190:bool)
                n2892 = local read "RATE (Hz)"() -> (w5199:dbl)
                n2893 = local read "SAMPLES"() -> (w5198:dbl)
                n2894 = Bundle("SET LAB01-1"=w5212, "SET LAB01-2"=w5211, "SET LAB02-1"=w5210, "SET LAB02-2"=w5209, "SET LAB03-1"=w5208, "SET LAB03-2"=w5207, "SET LAB04-1"=w5202, "SET LAB04-2"=w5203, "SET LAB05-1"=w5204, "SET LAB05-2"=w5205, "Network Directory"=w5206, "C drive data root dir"=w5200, "RATE (Hz)"=w5199, "SAMPLES"=w5198, "Select COM port"=w5197, "Temp Delay Lps"=w5196, "Temp Value"=w5195, "Fail Loops"=w5194, "Temp Test Cal"=w5193, "Amps Fail level"=w5192, "Mail Test File To:"=w5191, "Mail Test Fail"=w5190) -> (w5201:T24)  [unwired: 1 in]
              }
              frame #1 {
                n2895 = event shown="[1] \"SET LAB01-1\", \"SET LAB01-2\", \"SET LAB02-1\", \"SET LAB02-2\", \"SET LAB03-1\", \"SET LAB03-2\", \"SET LAB04-1\", \"SET LAB04-2\", \"SET LAB05-1\", \"SET LAB05-2\", \"Network Directory\", \"C drive data root dir\", \"RATE (Hz)\", \"SAMPLES\", \"Select COM port\", \"Temp Delay Lps\", \"Temp Value\", \"Fail Loops\", \"Temp Test Cal\", \"Amps Fail level\", \"Mail Test File To:\", \"Mail Test Fail\": Value Change" {
                  selector: _ -> [_ _ _]
                  dyn-events: _ -> [_ _ _]
                  timeout: 10.0 -> [_ _ _]
                  tunnel: w5215 -> [_ w5217 _]
                  tunnel: w5214 -> [_ w5218 _]
                  tunnel: w5213 -> [_ _ w5229]
                  event Timeout {
                    n2896 = event-data() -> ()  [unwired: 1 in, 3 out]
                  }
                  event "SET LAB01-2", "SET LAB02-1", "SET LAB02-2", "SET LAB03-1", "SET LAB03-2", "SET LAB04-1", "SET LAB04-2", "SET LAB05-1", "SET LAB05-2", "Network Directory", "C drive data root dir", "RATE (Hz)", "SAMPLES", "Select COM port", "Temp Delay Lps", "Temp Value", "Fail Loops", "Temp Test Cal", "Amps Fail level", "Mail Test File To:", "Mail Test Fail": Value Change {
                    n2897 = event-data() -> ()  [unwired: 1 in, 6 out]
                    n2898 = Open/Create/Replace File(file path (use dialog)=w5217, operation (0:open)=T18."replace or create") -> (refnum out=w5223:refnum<file>, error out=w5222:errorcluster)  [unwired: 4 in, 1 out]
                    n2899 = Write to Binary File(file (use dialog)=w5223, data=w5218, error in=w5222) -> (refnum out=w5221:refnum<file>, error out=w5220:errorcluster)  [unwired: 3 in, 1 out]
                    n2900 = Close File(refnum=w5221, error in=w5220) -> (error out=w5219:errorcluster)  [unwired: 1 out]
                    n2901 = local write "data file error"(w5219) -> ()
                  }
                  event "MAIL SETTINGS.OUT SERVER ADDRESS", "MAIL SETTINGS.FROM ACCOUNT", "MAIL SETTINGS.USER NAME", "MAIL SETTINGS.PASSWORD", "Auto Mail Send", "TO (string):": Value Change {
                    n2902 = event-data() -> ()  [unwired: 1 in, 6 out]
                    n2903 = local read "Auto Mail Send"() -> (w5226:bool)
                    n2904 = local read "MAIL SETTINGS"() -> (w5228:T8)
                    n2905 = local read "TO (string):"() -> (w5225:string)
                    n2906 = Open/Create/Replace File(file path (use dialog)=w5229, operation (0:open)=T18."replace or create") -> (refnum out=w5234:refnum<file>, error out=w5233:errorcluster)  [unwired: 4 in, 1 out]
                    n2907 = Bundle("MAIL SETTINGS"=w5228, "Auto Mail Send"=w5226, "TO (string):"=w5225) -> (w5227:T46)  [unwired: 1 in]
                    n2908 = Write to Binary File(file (use dialog)=w5234, data=w5227, error in=w5233) -> (refnum out=w5232:refnum<file>, error out=w5231:errorcluster)  [unwired: 3 in, 1 out]
                    n2909 = Close File(refnum=w5232, error in=w5231) -> (error out=w5230:errorcluster)  [unwired: 1 out]
                    n2910 = local write "data file error"(w5230) -> ()
                  }
                }
              }
            }
          }
          frame #19 {
            # "mail control"
            n2911 = local read "MAIL SETTINGS"() -> (w5251:T8)
            n2912 = local read "Auto Mail Send"() -> (w5237:bool)
            n2913 = Unbundle By Name(w5251) -> ("OUT SERVER ADDRESS"=w5250:string, "FROM ACCOUNT"=w5249:string, "TEST MAIL"=w5248:bool)
            n2914 = stacked-sequence {
              tunnel: "TO (string):" -> [_ w5290]
              tunnel: w5251 -> [w5256 w5289]
